vi "DataStream_Sort.vi"(4 "error in (no error)":errorcluster, 5 "data":u32[](array[numeric]), 6 "Mode (1)":u16=1, 7 "CH_enable":bool[](array[boolean])) -> (0 "error out":errorcluster, 1 "Channel Data":i32[][](array[numeric]), 2 "Channel count":i32, 3 "CH_enable dup":bool[](array[boolean]))   [LabVIEW 2010, in "lib1299.lvlib"]
doc: "This VI sorts the 32bit data stream from the data reader to individual arrays based on the number of active channels.\n\nInputs:\nCH_enable - boolean array of channels that are enabled (T = enabled)\ndata - 32bit data array from reader\nmode - mode for the plug-in (1)\n 0: dynamic mode\n 1: fixed mode - 8 channels\n 2: fixed mode - 4 channels\nerror in - error input cluster\n\nOutputs:\nChannel count - number of active channels\nCH_enable dup - duplicate of channel enable array\nChannel Data - 2D array of data (array of channel data arrays)\nError out - error output cluster"
uses:
  lib1299.lvlib
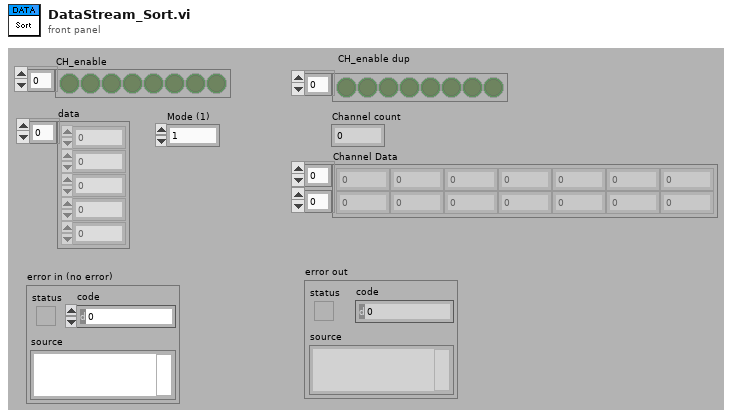
[diagram p1: front panel]
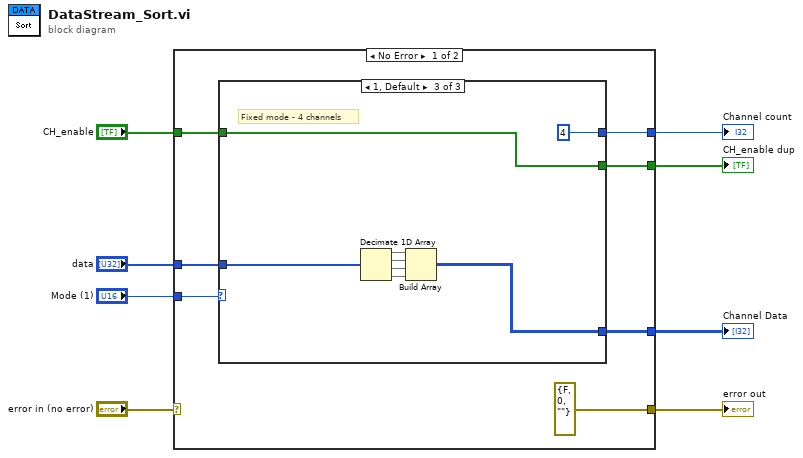
[diagram p0: block diagram]
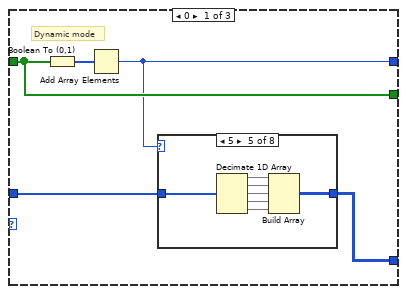
[diagram p2: hidden frame]
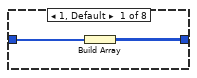
[diagram p3: hidden frame]
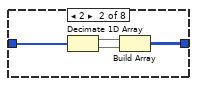
[diagram p4: hidden frame]
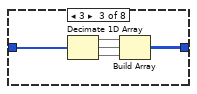
[diagram p5: hidden frame]
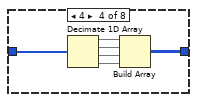
[diagram p6: hidden frame]
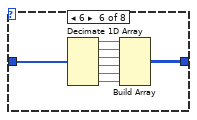
[diagram p7: hidden frame]
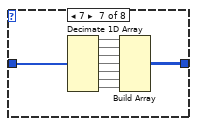
[diagram p8: hidden frame]
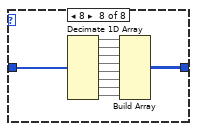
[diagram p9: hidden frame]
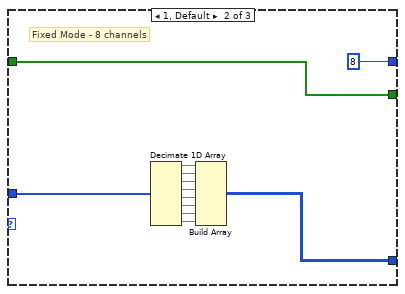
[diagram p10: hidden frame]
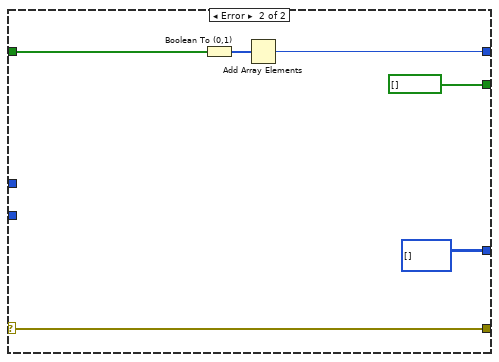
[diagram p11: hidden frame]
diagram:
  n1 = case shown="No Error" "error in (no error)" {
    selector: "error in (no error)" -> [_ w97]
    tunnel: "CH_enable" -> [w15 w95]
    tunnel: "Mode (1)" -> [w14 _]
    tunnel: "data" -> [w13 _]
    tunnel: [w12 w94] -> w5
    tunnel: [w11 u32[][] []] -> w4
    tunnel: [errorcluster {"status"=FALSE, "code"=0, "source"=""} ("error IO") w97] -> w2
    tunnel: [w9 bool[] [] ("CH_enable")] -> w1
    frame No Error {
      n2 = case shown="1, Default" w14 {
        tunnel: [w18 8 4] -> w12
        tunnel: w13 -> [w17 w82 w90]
        tunnel: w15 -> [w19 w72 w84]
        tunnel: [w16 w73 w85] -> w11
        tunnel: [w19 w72 w84] -> w9
        frame 0 {
          # "Dynamic mode"
          n3 = Boolean To (0,1)(Boolean=w19) -> (0, 1=w20:i16[])
          n4 = Add Array Elements(numeric array=w20) -> (sum=w18:i16)
          n5 = case shown="5" w18 {
            tunnel: w17 -> [w22 w26 w31 w37 w44 w52 w61 w71]
            tunnel: [w21 w23 w28 w34 w41 w49 w58 w68] -> w16
            frame 1, Default {
              n6 = Build Array(w22) -> (w21:u32[][])
            }
            frame 2 {
              n7 = Decimate 1D Array(w26) -> (w25:u32[], w24:u32[])
              n8 = Build Array(w25, w24) -> (w23:u32[][])
            }
            frame 3 {
              n9 = Decimate 1D Array(w31) -> (w30:u32[], w29:u32[], w27:u32[])
              n10 = Build Array(w30, w29, w27) -> (w28:u32[][])
            }
            frame 4 {
              n11 = Decimate 1D Array(w37) -> (w36:u32[], w35:u32[], w33:u32[], w32:u32[])
              n12 = Build Array(w36, w35, w33, w32) -> (w34:u32[][])
            }
            frame 5 {
              n13 = Decimate 1D Array(w44) -> (w43:u32[], w42:u32[], w40:u32[], w39:u32[], w38:u32[])
              n14 = Build Array(w43, w42, w40, w39, w38) -> (w41:u32[][])
            }
            frame 6 {
              n15 = Decimate 1D Array(w52) -> (w51:u32[], w50:u32[], w48:u32[], w47:u32[], w46:u32[], w45:u32[])
              n16 = Build Array(w51, w50, w48, w47, w46, w45) -> (w49:u32[][])
            }
            frame 7 {
              n17 = Decimate 1D Array(w61) -> (w60:u32[], w59:u32[], w57:u32[], w56:u32[], w55:u32[], w54:u32[], w53:u32[])
              n18 = Build Array(w60, w59, w57, w56, w55, w54, w53) -> (w58:u32[][])
            }
            frame 8 {
              n19 = Decimate 1D Array(w71) -> (w70:u32[], w69:u32[], w67:u32[], w66:u32[], w65:u32[], w64:u32[], w63:u32[], w62:u32[])
              n20 = Build Array(w70, w69, w67, w66, w65, w64, w63, w62) -> (w68:u32[][])
            }
          }
        }
        frame 1, Default {
          # "Fixed Mode - 8 channels"
          n21 = Decimate 1D Array(w82) -> (w81:u32[], w80:u32[], w79:u32[], w78:u32[], w77:u32[], w76:u32[], w75:u32[], w74:u32[])
          n22 = Build Array(w81, w80, w79, w78, w77, w76, w75, w74) -> (w73:u32[][])
        }
        frame 2 {
          # "Fixed mode - 4 channels"
          n23 = Decimate 1D Array(w90) -> (w89:u32[], w88:u32[], w87:u32[], w86:u32[])
          n24 = Build Array(w89, w88, w87, w86) -> (w85:u32[][])
        }
      }
    }
    frame Error {
      n25 = Boolean To (0,1)(Boolean=w95) -> (0, 1=w96:i16[])
      n26 = Add Array Elements(numeric array=w96) -> (sum=w94:i16)
    }
  }
  "CH_enable dup" <- w1
  "Channel Data" <- w4
  "Channel count" <- w5
  "error out" <- w2
